vi "cw_2_6.vi"() -> ()   [LabVIEW 2022 SP3]
panel:
  out "elapsed time [s]":ext
  in  "milliseconds to wait":u32
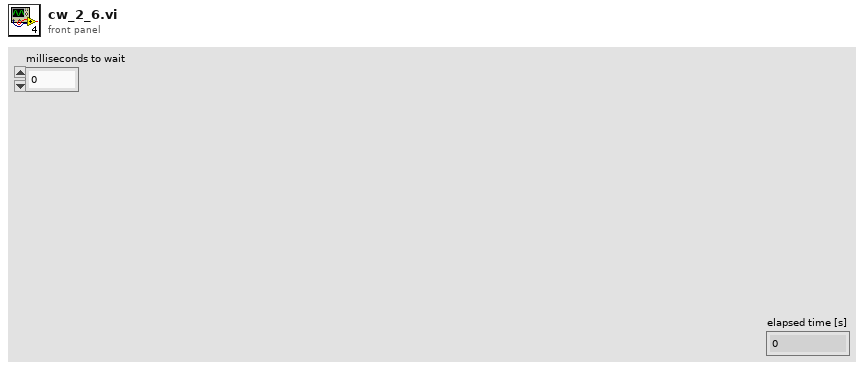
[diagram p1: front panel]
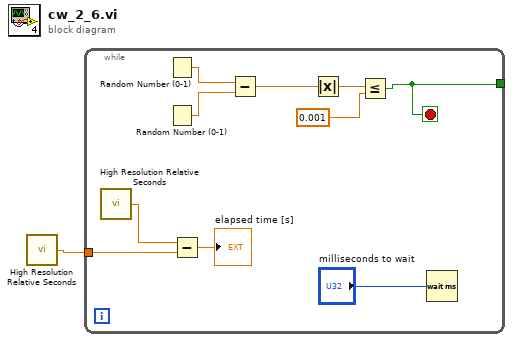
[diagram p0: block diagram]
diagram:
  n1 = call <vilib>:"High Resolution Relative Seconds.vi"() -> ("relative seconds"=w1:dbl)
  n2 = while {
    tunnel: [w5] -> _
    tunnel: w1 -> [w3]
    stop <- w5 stop-if-true
    n3 = call <vilib>:"High Resolution Relative Seconds.vi"() -> ("relative seconds"=w2:dbl)
    n4 = Random Number (0-1)() -> (number: 0 to 1=w11:dbl)
    n5 = Random Number (0-1)() -> (number: 0 to 1=w10:dbl)
    n6 = Subtract(x=w2, y=w3) -> (x-y=→"elapsed time [s]":dbl)
    n7 = Subtract(x=w11, y=w10) -> (x-y=w9:dbl)
    n8 = Absolute Value(x=w9) -> (abs(x)=w7:dbl)
    n9 = Less Or Equal?(x=w7, y=0.001) -> (x <= y?=w5:bool)
    n10 = Wait (ms)(milliseconds to wait="milliseconds to wait") -> ()  [unwired: 1 out]
  }
